vi "setProbeAttenuation.vi"(7 "Channel Name (0: Channel 1)":i32(ring) items=["Channel 1", "Channel 2", "Channel 3", "Channel 4"], 8 "error in (no error)":errorcluster, 10 "Probe Attenuation (1.0)":dbl=1.0, 11 "VISA resource name":refnum<visa-resource-name>) -> (0 "error out":errorcluster, 3 "VISA resource name out":refnum<visa-resource-name>)   [LabVIEW 2023, in "Keysight-DSQx3014T.lvlib"]
doc: "<b>Author:</b> Wolfgang Rominger\n<b>Description:</b> >>>> sets the probe attenuation >>>"
uses:
  Keysight-DSQx3014T.lvlib
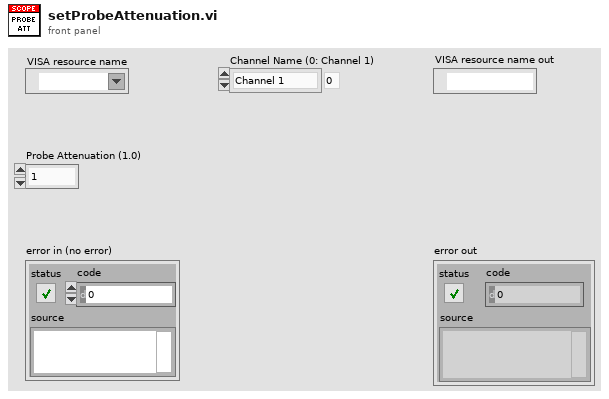
[diagram p1: front panel]
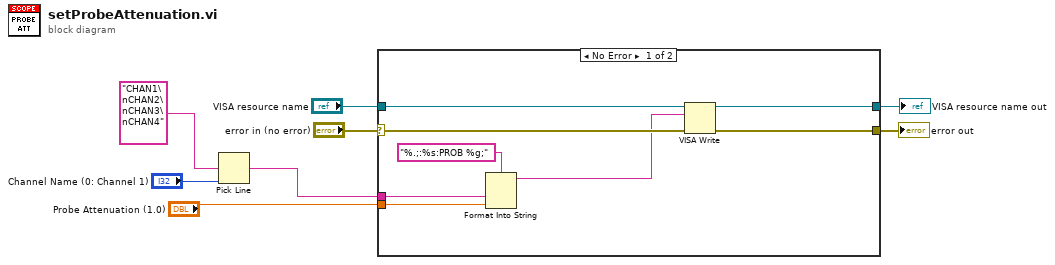
[diagram p0: block diagram]
diagram:
  n1 = Pick Line(multi-line string="CHAN1\nCHAN2\nCHAN3\nCHAN4", line index="Channel Name (0: Channel 1)") -> (output string=w2:string)  [unwired: 1 out]
  n2 = case shown="No Error" "error in (no error)" {
    selector: "error in (no error)" -> [w13 w18]
    tunnel: [w15 w17] -> w8
    tunnel: [w16 w18] -> w6
    tunnel: "VISA resource name" -> [w14 w17]
    tunnel: w2 -> [w10 _]
    tunnel: "Probe Attenuation (1.0)" -> [w9 _]
    frame No Error {
      n3 = Format Into String(format string="%.;:%s:PROB %g;", w10, w9) -> (resulting string=w11:string)  [unwired: 2 in, 1 out]
      n4 = VISA Write(VISA resource name=w14, write buffer=w11, error in (no error)=w13) -> (VISA resource name out=w15:refnum<visa-resource-name>, error out=w16:errorcluster)  [unwired: 1 out]
    }
    frame Error {
    }
  }
  "VISA resource name out" <- w8
  "error out" <- w6
